vi "_Remote Updata Parameter.vi"(1 "error in":errorcluster, 2 "Parameters":T1[](array[typedef])) -> (0 "error out":errorcluster)   [LabVIEW 2015]
uses:
  Type/_RT Active Ch.ctl
  Type/_RT Command.ctl
  Type/_RT Parameter.ctl
  Type/_RT Expt.ctl
  Type/_Run Mode.ctl
  Type/_RT Mass Range.ctl
  Type/_RT Res Type.ctl
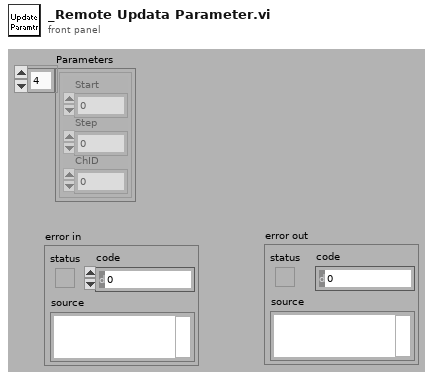
[diagram p1: front panel]
types:
  T1 = typedef "_RT Active Ch.ctl" = cluster{"Start":i32, "Step":i32, "ChID":i32}
  T2 = typedef "_RT Expt.ctl" = cluster{"StartT(mS)":i32, "#Cycles":i32, "Scan Type":T3, "PauseT(uS)":i32, "Polarity":u8, "DelayT(mS)":i32, "Active Ch":T1[], "Mass Range":T4[]}
  T3 = typedef "_Run Mode.ctl" = enum16{"MRM (Q1/Q2)", "Q1 Scan", "Q1 SRM", "Q2 Scan", "Q2 SRM", "Product Scan", "Precursor Scan", "Neutral Loss", "Neutral Gain"}
  T4 = typedef "_RT Mass Range.ctl" = cluster{"Steps":i32, "Dwell(uS)":i32, "Resolution Type":T5, "Ramping Ch":T1[]}
  T5 = typedef "_RT Res Type.ctl" = u16
  T6 = typedef "_RT Parameter.ctl" = cluster{"RunMode":i32, "Initial Ch":T1[], "Sync":u8, "Expt":T2[], "EqTime(mS)":i32}
  T7 = typedef "_RT Command.ctl" = enum16{"Start", "Stop", "Runtime Update", "Get Data", "Get Info", "Get Status", "Get Param", "Get Config", "Get Table", "Read ADC", "Set Oscillator", "Update Config", "Update Table", "Set All Pol", "Set Pol and DC", "Set Max Mass", "Toggle RP", "Toggle EL", "Set PIC", "Initialize Turbo", "Send Turbo Comm", "Close Turbo", "P1", "P2", "P3", "Send Serial", "Set LC Out", "Get LC In", "Read VAC", "Test Table", "Toggle Power", "Get Startup", "Set Startup", "Get ADC Table", "Set ADC Table", "Get Brief Status", "Get Detail Status", "Auxiliary Update", "Set CC Logics", "Set CC Input Logics", "Ignore Error"}
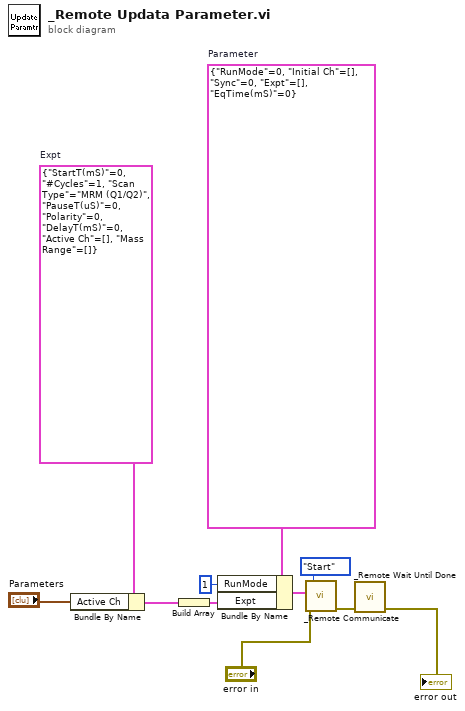
[diagram p0: block diagram]
diagram:
  w8 = T2 {"StartT(mS)"=0, "#Cycles"=1, "Scan Type"=enum."MRM (Q1/Q2)", "PauseT(uS)"=0, "Polarity"=0, "DelayT(mS)"=0, "Active Ch"=[], "Mass Range"=[]}  # Expt
  w5 = T6 {"RunMode"=0, "Initial Ch"=[], "Sync"=0, "Expt"=[], "EqTime(mS)"=0}  # Parameter
  n1 = Bundle By Name(cluster=w8, "Active Ch"="Parameters") -> (w9:T2)
  n2 = Build Array(w9) -> (w10:T2[])
  n3 = Bundle By Name(cluster=w5, "RunMode"=1, "Expt"=w10) -> (w6:T6)
  n4 = call "_Remote Communicate.vi"("error in (no error)"="error in", "Parameter"=w6, "Command"=_RT_Command."Start") -> ("error out"=w4:errorcluster)  [unwired: 3 in, 3 out]
  n5 = call "_Remote Wait Until Done.vi"("error IO"=w4) -> ("error out"=→"error out":errorcluster)  [unwired: 1 in, 1 out]
